vi "SystemCheck.vi"() -> ()   [LabVIEW 2021]
uses:
  Motion/EnableSingle.vi
panel:
  out "Axes":i32
  out "SMC version":string
  out "error out":errorcluster
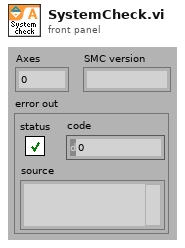
[diagram p1: front panel]
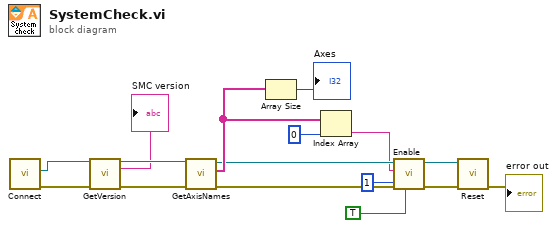
[diagram p0: block diagram]
diagram:
  n1 = call "Connect.vi"() -> ("error out"=w16:errorcluster, "controller"=w15:refnum<k24>)  [unwired: 10 in]
  n2 = call "GetVersion.vi"("controller in"=w15, "error in (no error)"=w16) -> ("controller out"=w14:refnum<k24>, "SMC version"=→"SMC version":string, "error out"=w13:errorcluster)  [unwired: 11 in]
  n3 = call "GetAxisNames.vi"("error in (no error)"=w13, "controller in"=w14) -> ("error out"=w5:errorcluster, "axis names"=w9:string[], "controller out"=w7:refnum<k24>)  [unwired: 7 in]
  n4 = Array Size(array=w9) -> (size(s)=→"Axes":i32)
  n5 = Index Array(array=w9, index=0) -> (element=w3:string)
  n6 = call-poly "Enable.vi"("return immediately"=TRUE, "error in (no error)"=w5, "taskId"=1 ("taskNumber"), "axis name"=w3, "controller in"=w7) -> ("error out"=w4:errorcluster, "controller out"=w6:refnum<k24>)  [unwired: 5 in]
  n7 = call "Reset.vi"("error in (no error)"=w4, "controller in"=w6) -> ("error out"=→"error out":errorcluster)  [unwired: 8 in, 1 out]
